vi "ES2 Main.vi"(10 "Data Type DVRs":T1, 11 "Config Folder":path) -> ()   [LabVIEW 2018]
uses:
  <vilib>/ORNL/CSEISMIC DDS/CSEISMIC DDS Base/Data Types/Controls/DeviceID.ctl
  Controls/DDS State.ctl
  Controls/Data Type DVRs.ctl
  Controls/Generation Mode Loop Selector.ctl
  <vilib>/ORNL/CSEISMIC DDS/CSEISMIC DDS Base/Data Types/DER_setGenerationMode.ctl
  <vilib>/ORNL/CSEISMIC DDS/CSEISMIC DDS Base/Data Types/Controls/Generation Mode.ctl
  Controls/GenerationMode.ctl
  <vilib>/ORNL/CSEISMIC DDS/CSEISMIC DDS Base/Data Types/IED_Status.ctl
  <vilib>/ORNL/CSEISMIC DDS/CSEISMIC DDS Base/Data Types/Controls/Timestamp.ctl
  <vilib>/ORNL/CSEISMIC DDS/CSEISMIC DDS Base/Data Types/DER_Control.ctl
  <vilib>/ORNL/CSEISMIC DDS/CSEISMIC DDS Base/Data Types/DER_SetPointP.ctl
  <vilib>/ORNL/CSEISMIC DDS/CSEISMIC DDS Base/Data Types/DER_SetPointQ.ctl
  <vilib>/ORNL/CSEISMIC DDS/CSEISMIC DDS Base/Data Types/DER_SetPointV.ctl
  <vilib>/ORNL/CSEISMIC DDS/CSEISMIC DDS Base/Data Types/DER_VF.ctl
  <vilib>/ORNL/CSEISMIC DDS/CSEISMIC DDS Base/Data Types/DER_SetPointF.ctl
  <vilib>/ORNL/CSEISMIC DDS/CSEISMIC DDS Base/Data Types/DER_Measurement.ctl
  <vilib>/ORNL/CSEISMIC DDS/CSEISMIC DDS Base/Data Types/DER_Status.ctl
  <vilib>/ORNL/CSEISMIC DDS/CSEISMIC DDS Base/Data Types/Controls/DroopCurve.ctl
  <vilib>/ORNL/CSEISMIC DDS/CSEISMIC DDS Base/Data Types/ES_Measurement.ctl
  c0909f76-96e0-496f-a6f7-ac9c3abfbcaa.vi
  7c59bdfa-a6d0-42ea-a36a-6a540bb37f3e.vi
  e95f3c18-e29d-40e4-94d7-6429cff7ece6.vi
  5e6c5b3f-77aa-4a8f-ba55-705d5b229056.vi
  7d30dc78-1fe7-43d0-be68-14ef1da03709.vi
  d3906dff-0d56-43f1-806b-b312a818046b.vi
  60710d3d-d05d-4e06-abc4-5833922697d4.vi
  d723711c-90b5-43fd-9837-430fe65d8763.vi
  2b29db2b-b629-43ef-99c9-7f779e92d8e6.vi
  fb202ae5-af77-46d5-8a34-636558cc811c.vi
  de1367b4-29ab-415d-92d0-7fa0fc6667ea.vi
  a8c78b73-a0ab-4721-a181-3ce0dcbdf431.vi
  9b782105-9e9e-450c-bef0-451d1281a5e4.vi
  04e9c7aa-85a8-4273-86f5-9355a9113040.vi
  f60448c4-0b4d-4df0-bc80-4b02817c393f.vi
  ae97810f-c92e-4387-8c39-39f975af07db.vi
  Global Variables/Stop (Global).vi
  Global Variables/Measurements (Global).vi
  Global Variables/DDS States (Global).vi
  <vilib>/ORNL/CSEISMIC DDS/CSEISMIC DDS Base/CSEISMIC DDS.lvclass
panel:
  out "P_ref":sgl
  out "Q_ref":sgl
  out "P_meas":sgl
  out "Vf Control":bool
  out "Q_meas":sgl
  out "f_islanded":fxp<+,20,6>
  out "Vq_ref":sgl
  out "5038 Count":u32
  out "Is VF Device?":bool
  in  "Ramp Rate (W)":sgl=5000.0
  out "MicrogridID":u8
  out "Error in DDS Loop":bool
  out "DDS Loop error out":errorcluster
  out "DDS State":T2=enum."Shutdown"
  out "DDS loop time":u32=103
  out "DDS Indicators":T3
  out "Error in Generation Mode Loop":bool
  out "error out GenMode Loop":errorcluster
  out "DDS state m/c loop time":u32=100
  out "DeviceID":T4
  out "Enable INV A":bool
  out "SOC":dbl
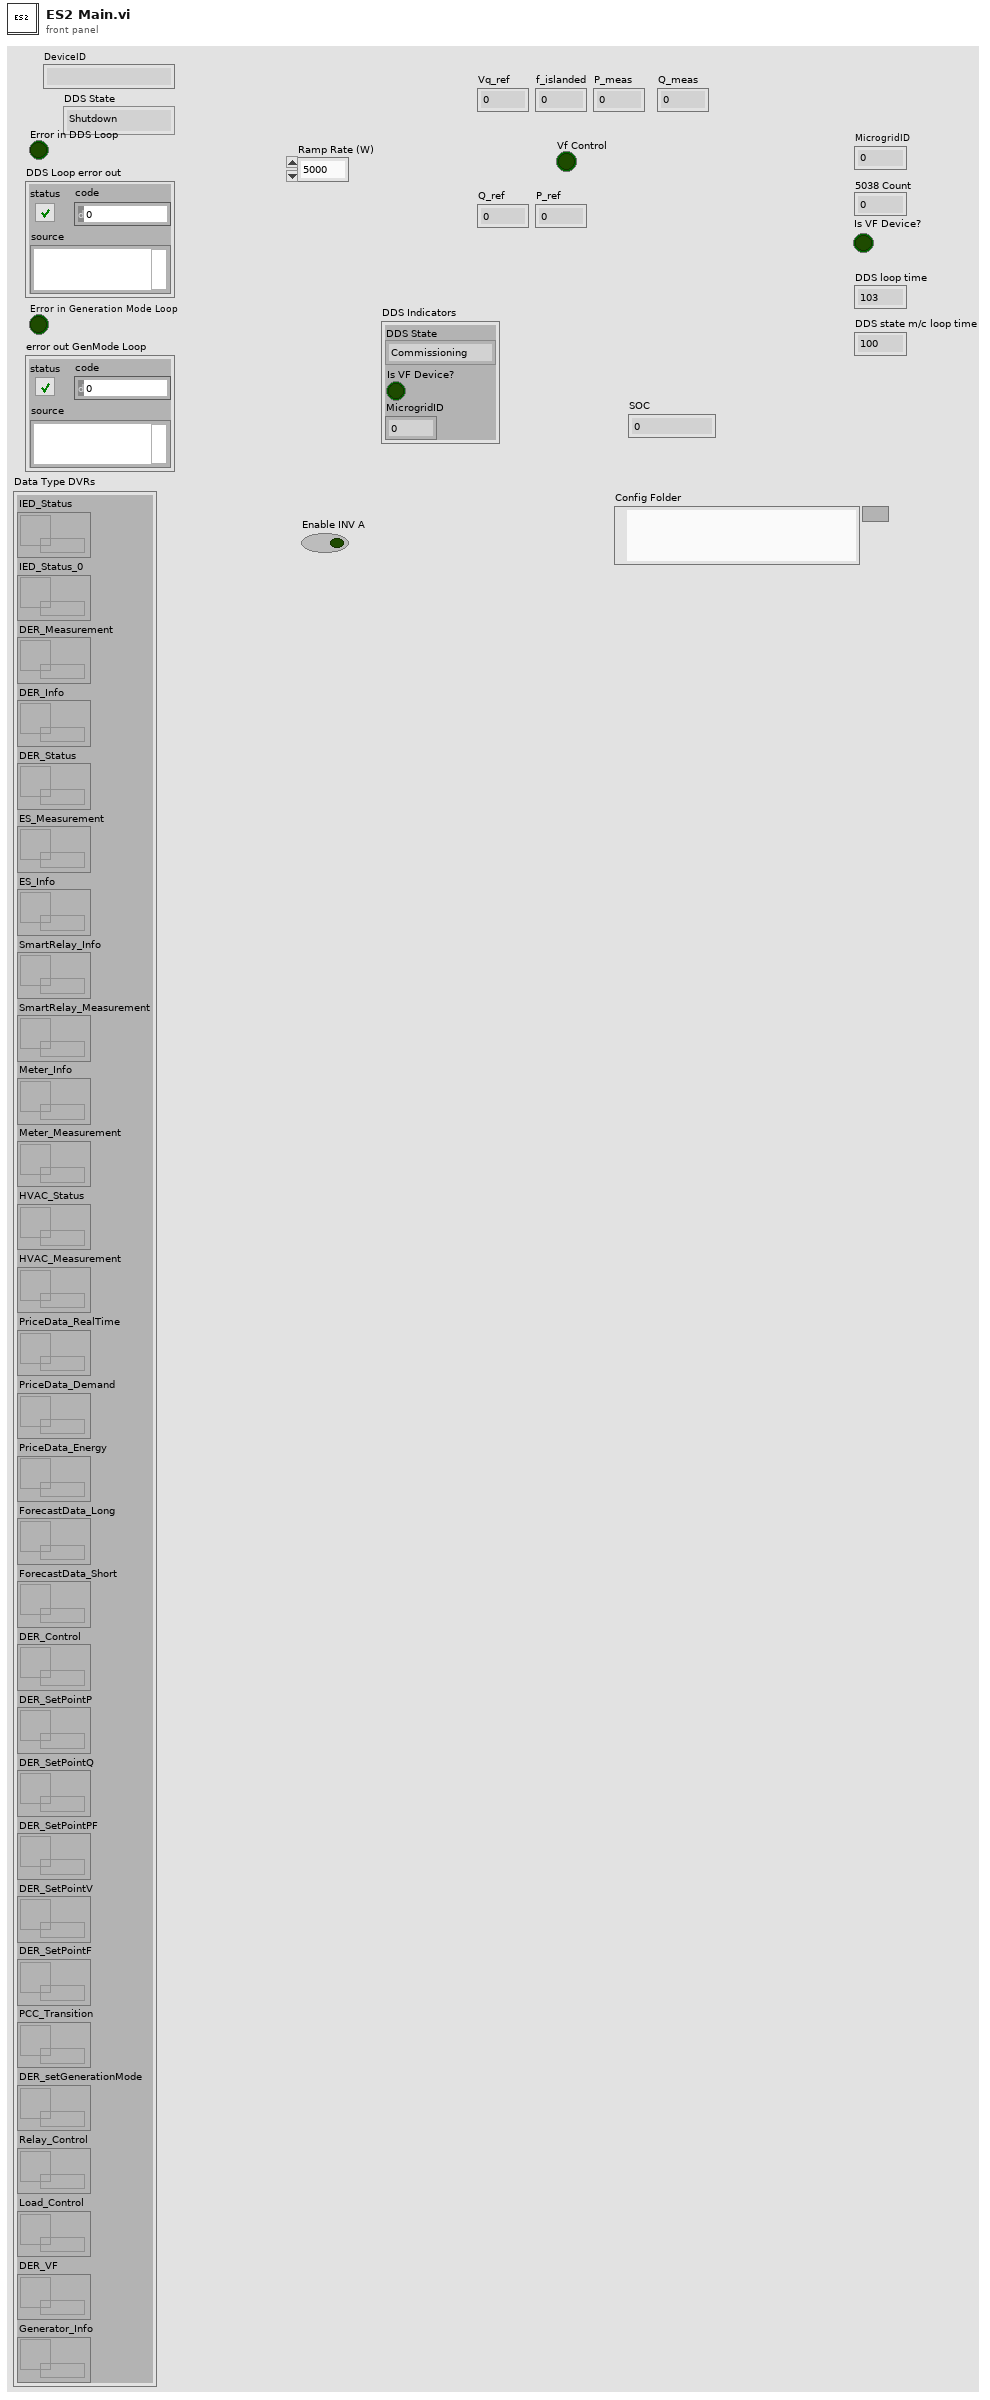
[diagram p1: front panel]
types:
  T1 = typedef "Data Type DVRs.ctl" = cluster{"IED_Status":refnum<data-value>, "IED_Status_0":refnum<data-value>, "DER_Measurement":refnum<data-value>, "DER_Info":refnum<data-value>, "DER_Status":refnum<data-value>, "ES_Measurement":refnum<data-value>, "ES_Info":refnum<data-value>, "SmartRelay_Info":refnum<data-value>, "SmartRelay_Measurement":refnum<data-value>, "Meter_Info":refnum<data-value>, "Meter_Measurement":refnum<data-value>, "HVAC_Status":refnum<data-value>, "HVAC_Measurement":refnum<data-value>, "PriceData_RealTime":refnum<data-value>, "PriceData_Demand":refnum<data-value>, "PriceData_Energy":refnum<data-value>, "ForecastData_Long":refnum<data-value>, "ForecastData_Short":refnum<data-value>, "DER_Control":refnum<data-value>, "DER_SetPointP":refnum<data-value>, "DER_SetPointQ":refnum<data-value>, "DER_SetPointPF":refnum<data-value>, "DER_SetPointV":refnum<data-value>, "DER_SetPointF":refnum<data-value>, "PCC_Transition":refnum<data-value>, "DER_setGenerationMode":refnum<data-value>, "Relay_Control":refnum<data-value>, "Load_Control":refnum<data-value>, "DER_VF":refnum<data-value>, "Generator_Info":refnum<data-value>}
  T2 = typedef "DDS State.ctl" = enum16{"Commissioning", "CheckID", "InitDDS", "ReadDDS", "WriteDDS", "CheckClose", "Close", "Shutdown"}
  T3 = cluster{"DDS State":T2, "Is VF Device?":bool, "MicrogridID":u8}
  T4 = typedef "CSEISMIC DDS.lvlib/CSEISMIC DDS.lvclass/DeviceID.ctl" = string
  T5 = typedef "Generation Mode Loop Selector.ctl" = enum16{"Commissioning", "Start", "Active", "VF Device", "Hold", "Close References", "Shutdown"}
  T6 = typedef "Scaling Coefficients Cluster.ctl" = cluster{"Measurements":T7, "Setpoints":T8}
  T7 = typedef "Scaling Coefficients Measurements.ctl" = cluster{"Current":dbl, "Voltage":dbl, "Real Power":dbl, "Reactive Power":dbl, "SOC":dbl}
  T8 = typedef "Scaling Coefficients Setpoints.ctl" = cluster{"Voltage":dbl, "Frequency":dbl, "Real Power":dbl, "Reactive Power":dbl}
  T9 = typedef "CSEISMIC DDS.lvlib/CSEISMIC DDS.lvclass/DER_Info.ctl" = cluster{"DeviceID":T4, "LineConfig":u8[], "NominalVoltage(V)":dbl, "PowerRating(kVA)":dbl, "VFControl":bool, "PControl":bool, "QControl":bool, "PFControl":bool, "PVControl":bool, "Droop":bool, "DroopConfigurable":bool, "Unbalanced":bool}
  T10 = typedef "CSEISMIC DDS.lvlib/CSEISMIC DDS.lvclass/ES_Info.ctl" = cluster{"DeviceID":T4, "EnergyRating (kWh)":dbl, "RampRate (kW/s)":dbl, "MaxPowerFactorLeading":dbl, "MaxPowerFactorLagging":dbl, "ChargingEfficiencyCurve":T11, "DischargingEfficiencyCurve":T11, "MinSOC (%)":dbl, "MaxSOC (%)":dbl}
  T11 = typedef "CSEISMIC DDS.lvlib/CSEISMIC DDS.lvclass/EfficiencyCurve.ctl" = cluster{"Power (kW)":dbl[], "Efficiency (%)":dbl[]}
  T12 = typedef "CSEISMIC DDS.lvlib/CSEISMIC DDS.lvclass/DER_setGenerationMode.ctl" = cluster{"DeviceID":T4, "Mode":T13}
  T13 = typedef "CSEISMIC DDS.lvlib/CSEISMIC DDS.lvclass/Generation Mode.ctl" = enum32{"Invalid", "PQ", "Droop", "PV", "PF", "VF"}
  T14 = typedef "GenerationMode.ctl" = enum32{"Invalid", "PQ", "Droop", "PV", "PF", "VF"}
  T15 = typedef "CSEISMIC DDS.lvlib/CSEISMIC DDS.lvclass/Timestamp.ctl" = cluster{"Seconds":u64, "Remainder":u64}
  T16 = typedef "CSEISMIC DDS.lvlib/CSEISMIC DDS.lvclass/IED_Status.ctl" = cluster{"DeviceID":T4, "Timestamp":T15, "MicrogridID":u8, "Active":bool, "Inactive":bool, "Error":i32, "Fault":bool, "ErrorString":string}
  T17 = typedef "CSEISMIC DDS.lvlib/CSEISMIC DDS.lvclass/DER_SetPointF.ctl" = cluster{"DeviceID":T4, "Frequency (Hz)":dbl}
  T18 = typedef "CSEISMIC DDS.lvlib/CSEISMIC DDS.lvclass/DER_VF.ctl" = cluster{"DeviceID":T4}
  T19 = typedef "CSEISMIC DDS.lvlib/CSEISMIC DDS.lvclass/DER_SetPointV.ctl" = cluster{"DeviceID":T4, "Voltage (V)":dbl}
  T20 = typedef "CSEISMIC DDS.lvlib/CSEISMIC DDS.lvclass/DER_SetPointQ.ctl" = cluster{"DeviceID":T4, "ReactivePower (kVAR)":dbl[]}
  T21 = typedef "CSEISMIC DDS.lvlib/CSEISMIC DDS.lvclass/DER_SetPointP.ctl" = cluster{"DeviceID":T4, "RealPower (kW)":dbl[]}
  T22 = typedef "CSEISMIC DDS.lvlib/CSEISMIC DDS.lvclass/DER_Control.ctl" = cluster{"DeviceID":T4, "Activate":bool, "Deactivate":bool}
  T23 = typedef "CSEISMIC DDS.lvlib/CSEISMIC DDS.lvclass/ES_Measurement.ctl" = cluster{"DeviceID":T4, "SOC (%)":dbl}
  T24 = typedef "CSEISMIC DDS.lvlib/CSEISMIC DDS.lvclass/DER_Status.ctl" = cluster{"DeviceID":T4, "VFControl":bool, "PControl":bool, "QControl":bool, "PFControl":bool, "PVControl":bool, "Droop":bool, "Unbalanced":bool, "MicrogridVF":bool, "RealDroop(kW)":T25, "ReactiveDroop(kVar)":T25}
  T25 = typedef "CSEISMIC DDS.lvlib/CSEISMIC DDS.lvclass/DroopCurve.ctl" = cluster{"XMin":dbl, "XMax":dbl, "YMin":dbl, "YMax":dbl}
  T26 = typedef "CSEISMIC DDS.lvlib/CSEISMIC DDS.lvclass/DER_Measurement.ctl" = cluster{"DeviceID":T4, "Voltage":dbl[], "Current":dbl[], "RealPower":dbl[], "ReactivePower":dbl[], "LineConfig":u8[], "Frequency":dbl}
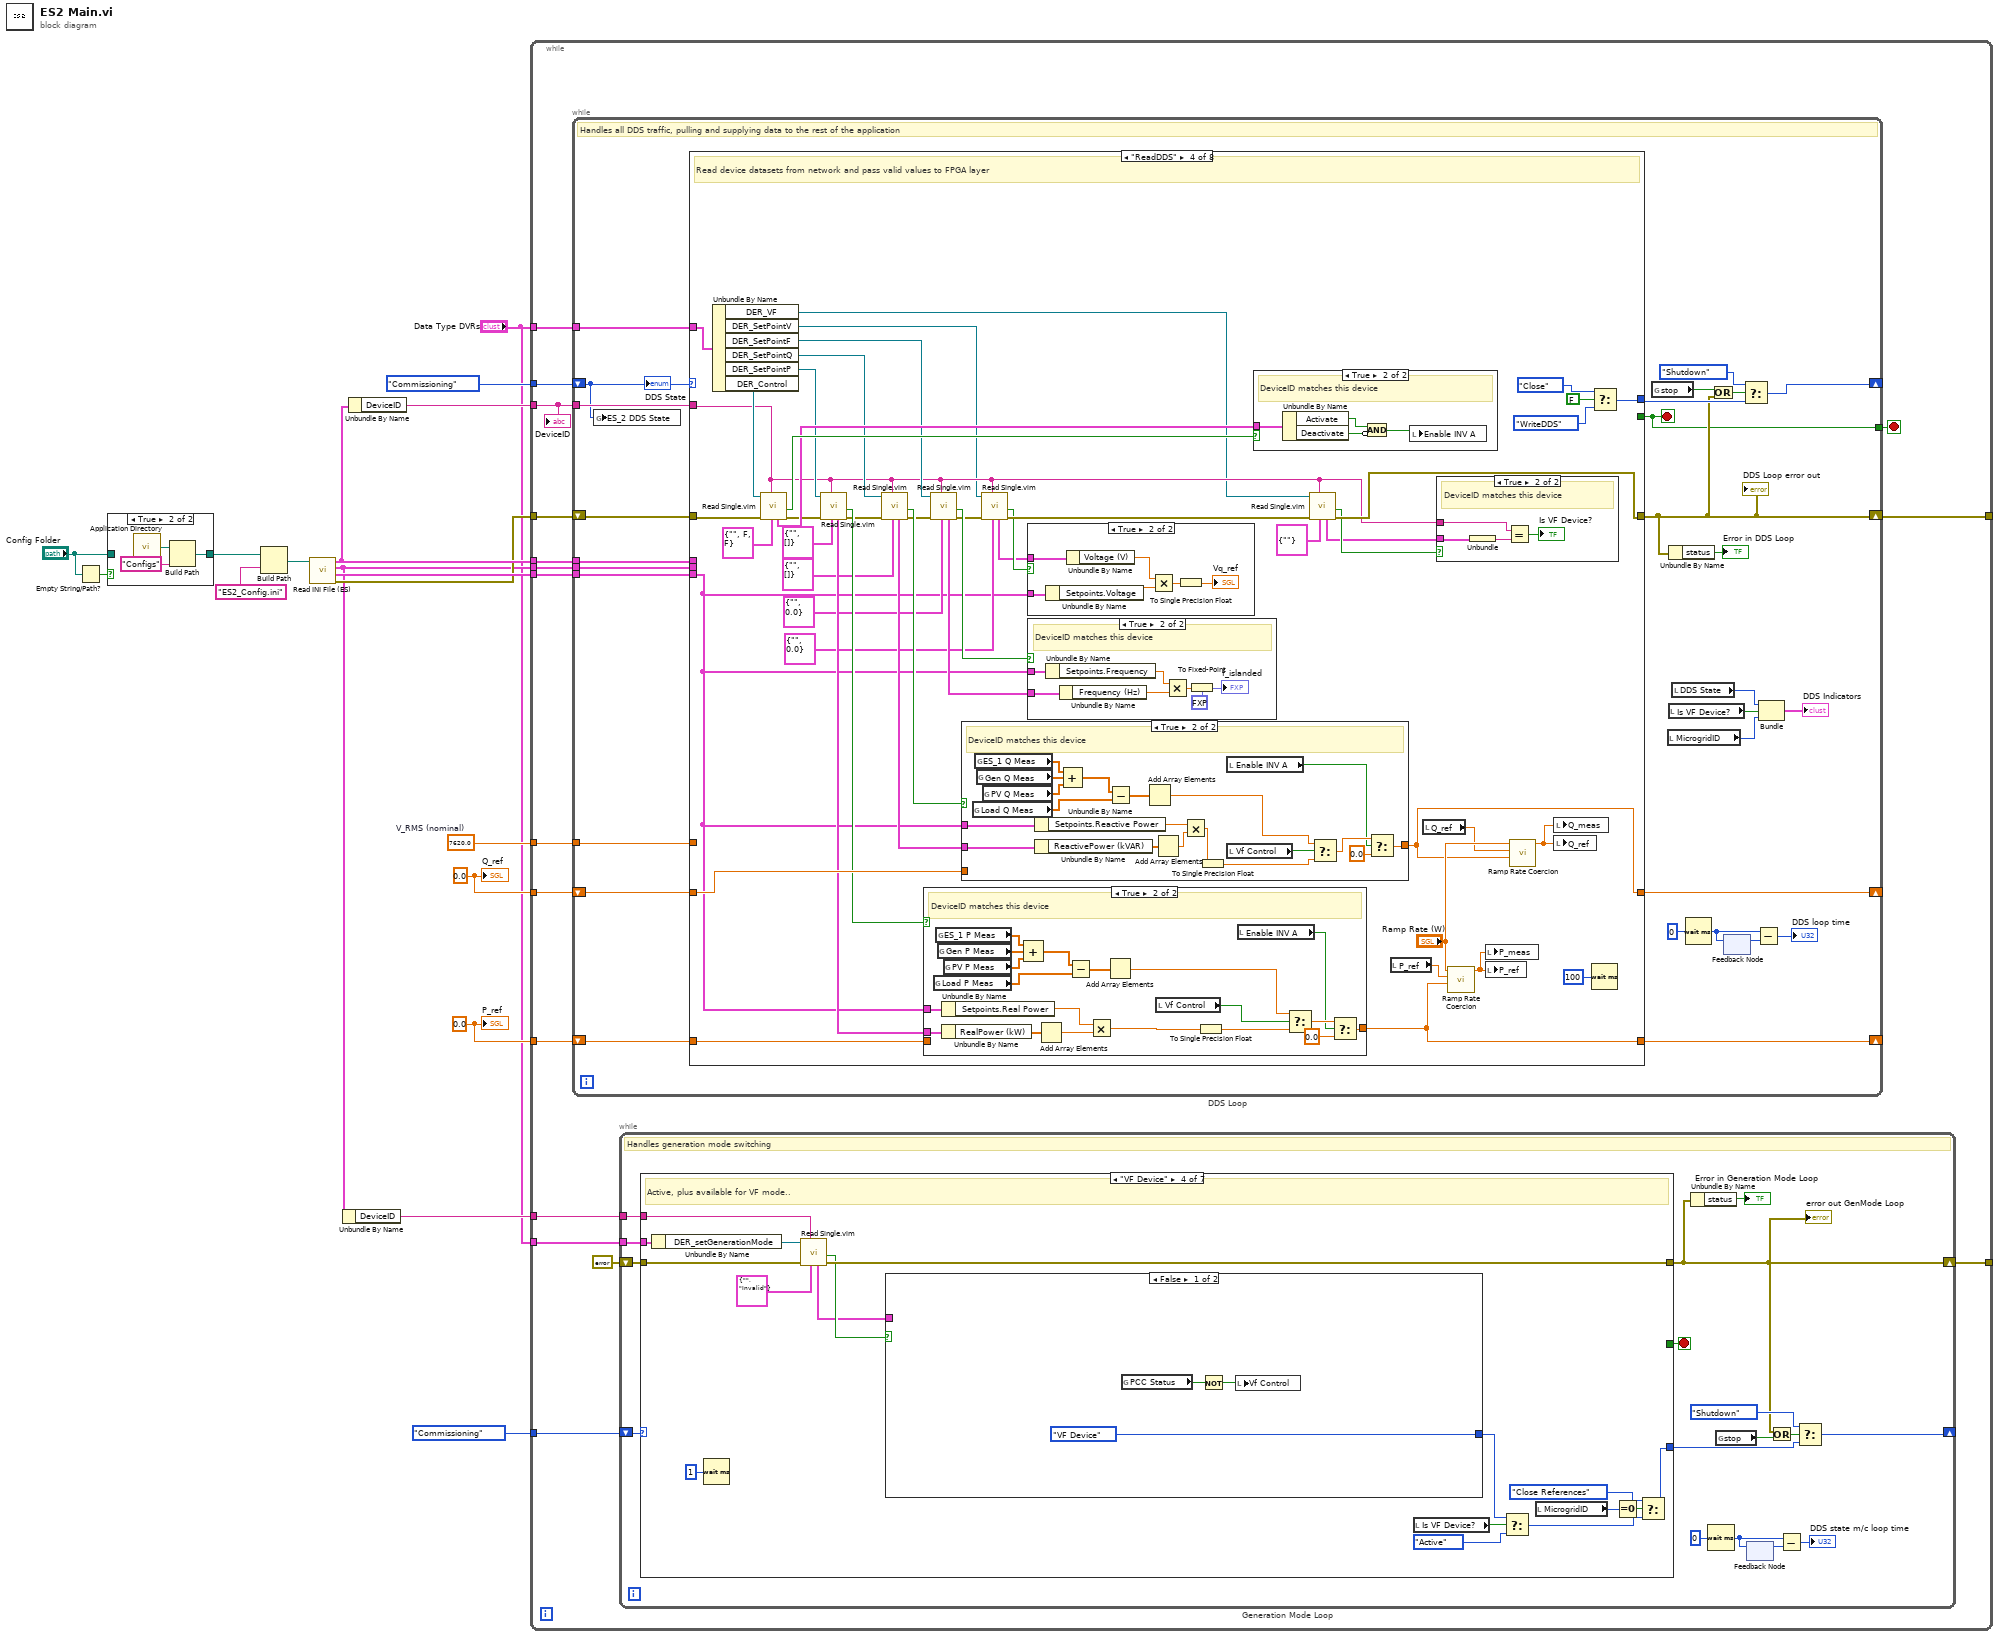
[diagram p0: block diagram]
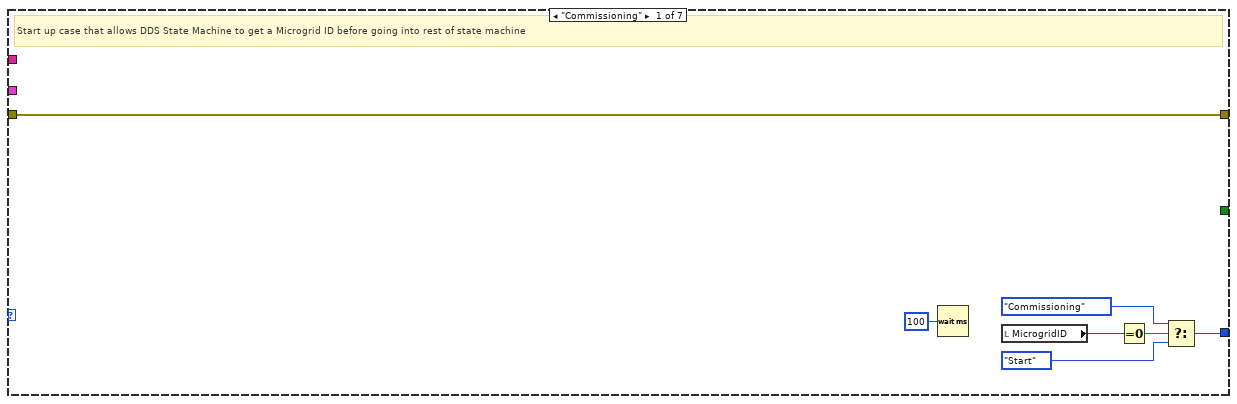
[diagram p2: hidden frame]
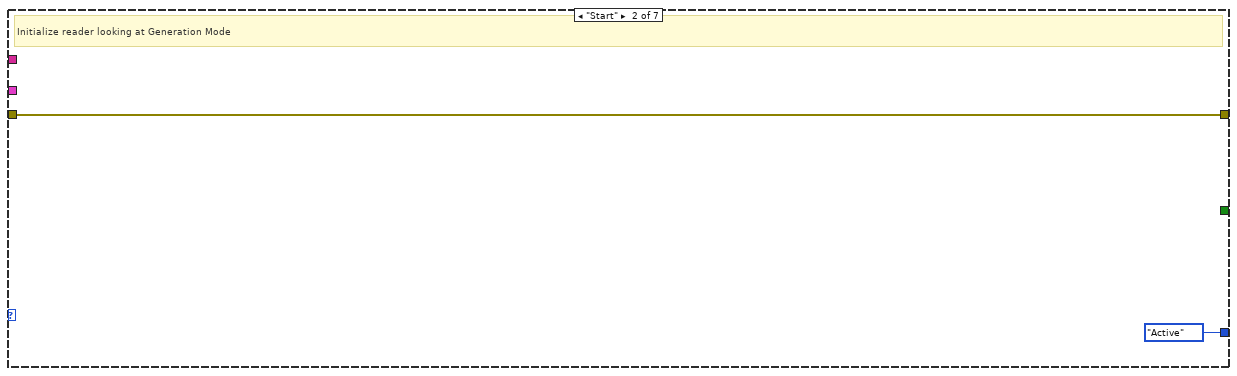
[diagram p3: hidden frame]
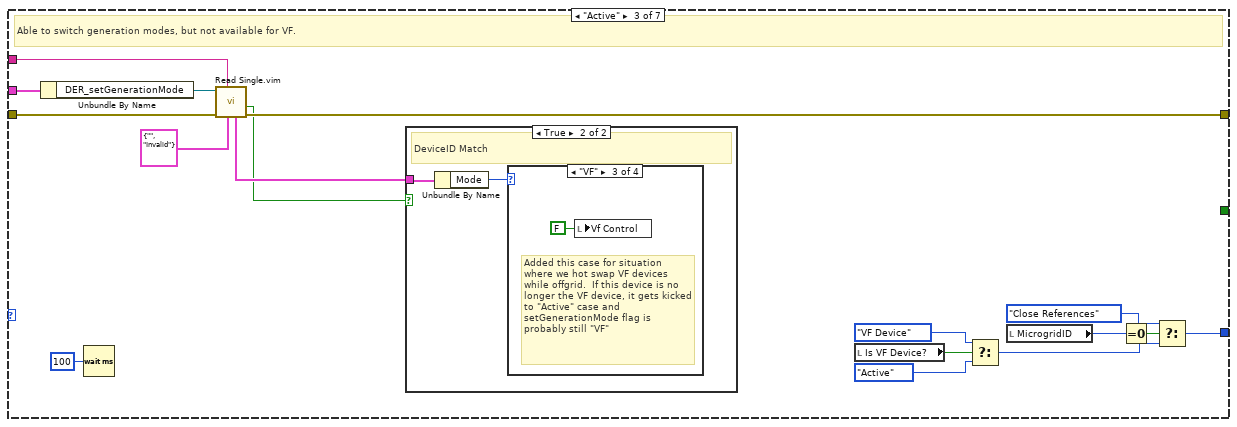
[diagram p4: hidden frame]
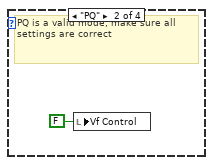
[diagram p7: hidden frame]
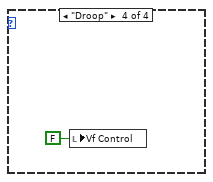
[diagram p8: hidden frame]
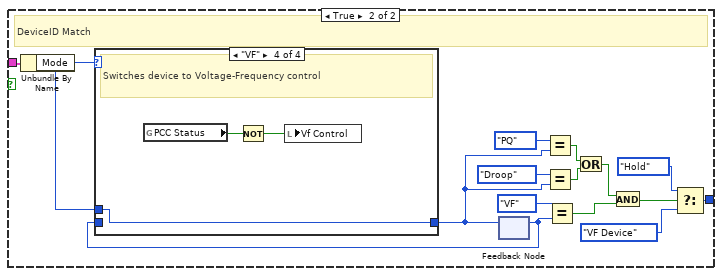
[diagram p9: hidden frame]
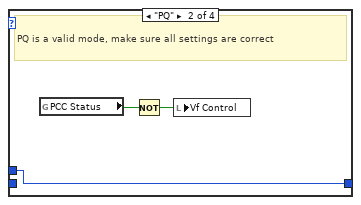
[diagram p11: hidden frame]
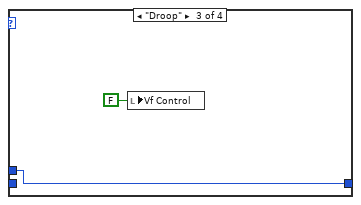
[diagram p12: hidden frame]
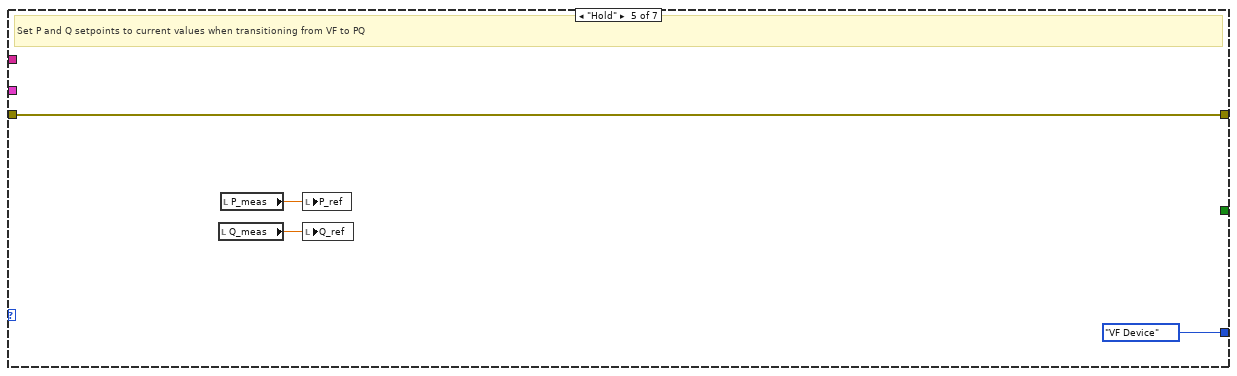
[diagram p13: hidden frame]
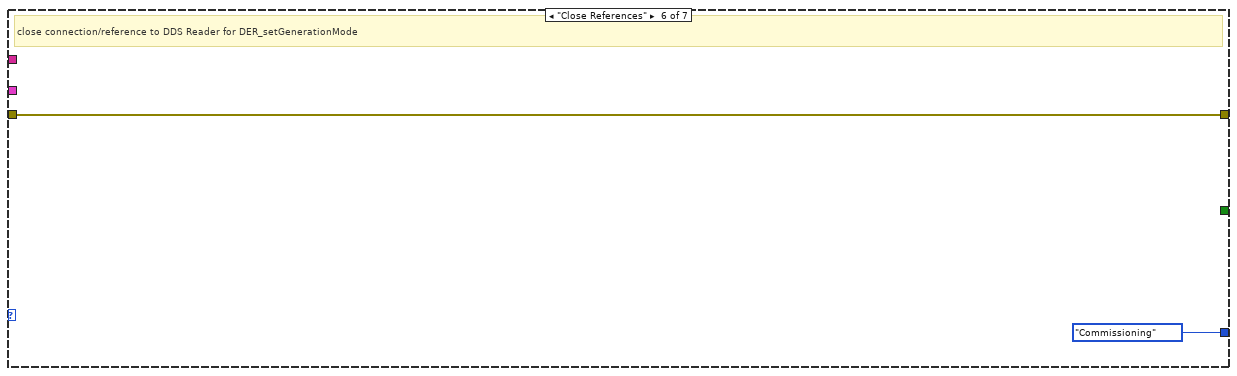
[diagram p14: hidden frame]
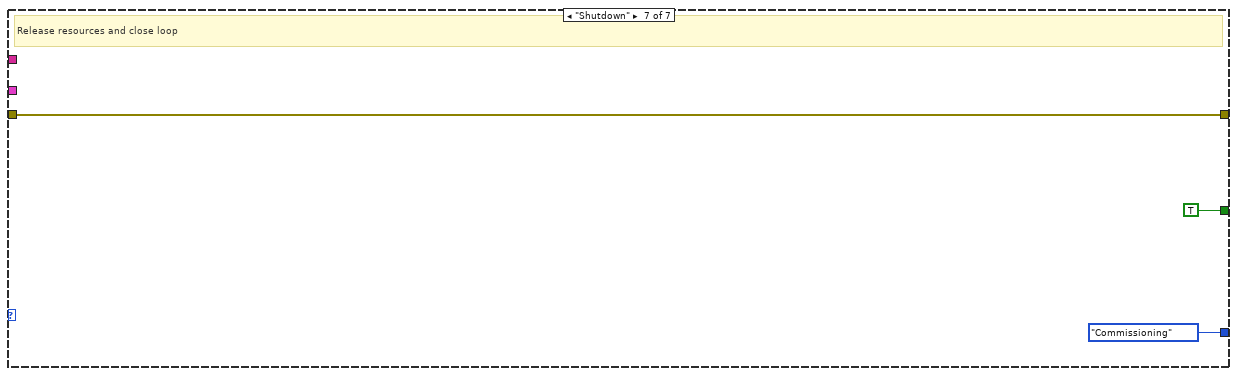
[diagram p15: hidden frame]
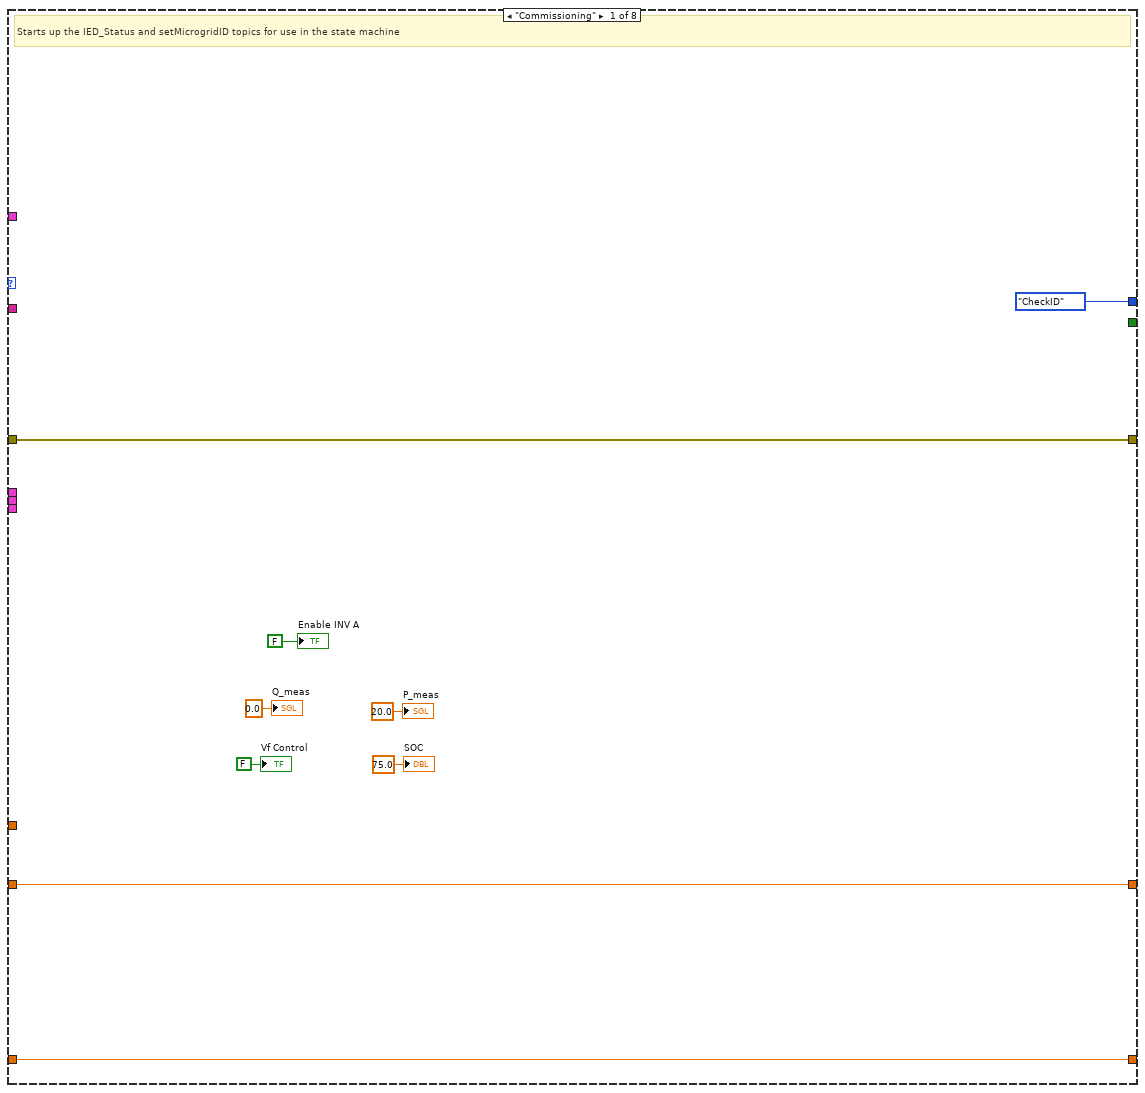
[diagram p16: hidden frame]
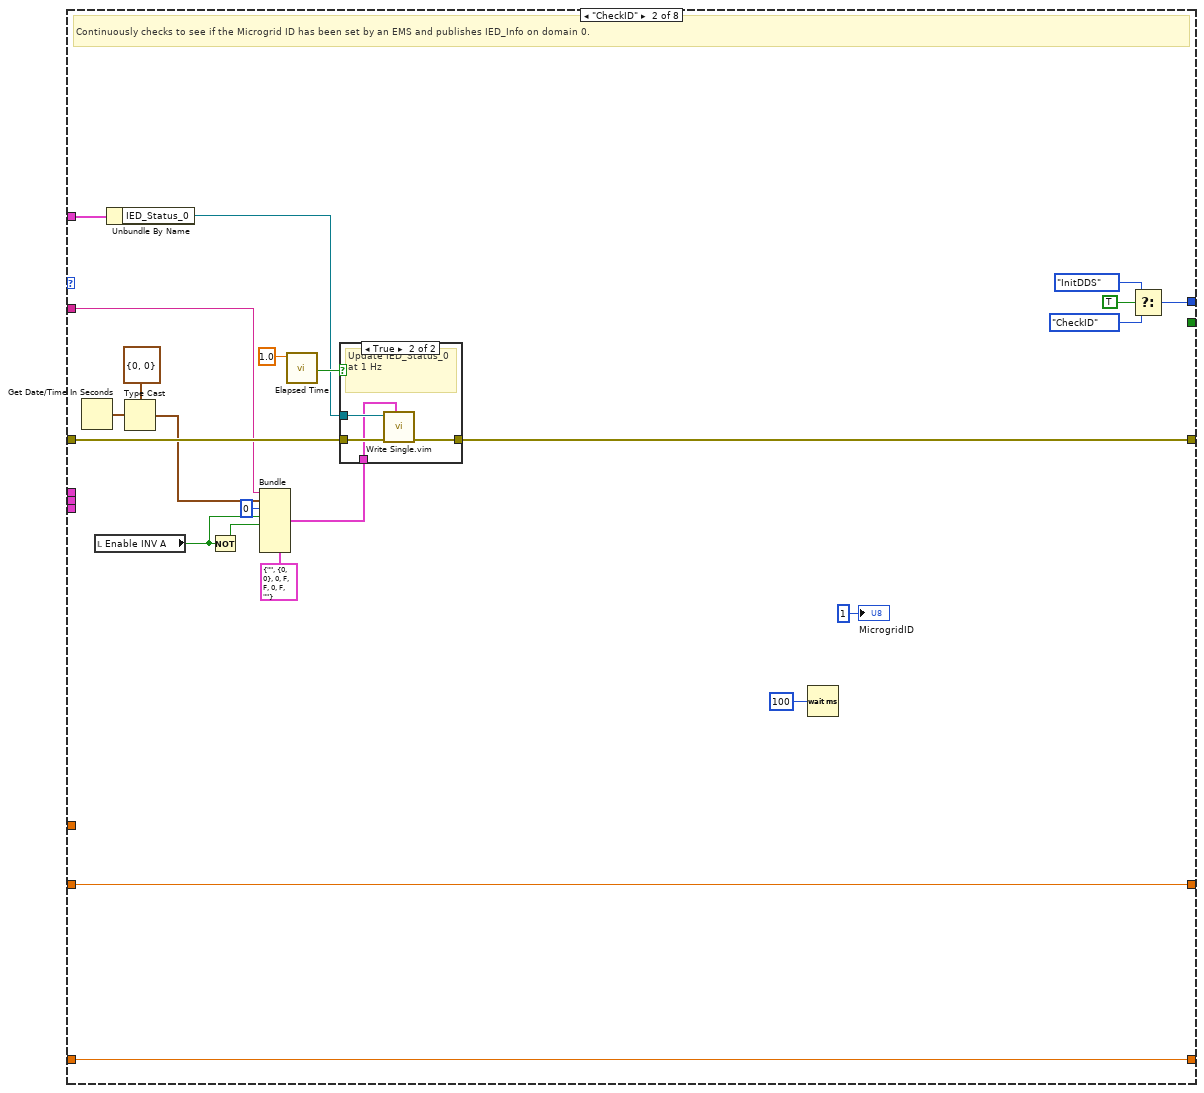
[diagram p17: hidden frame]
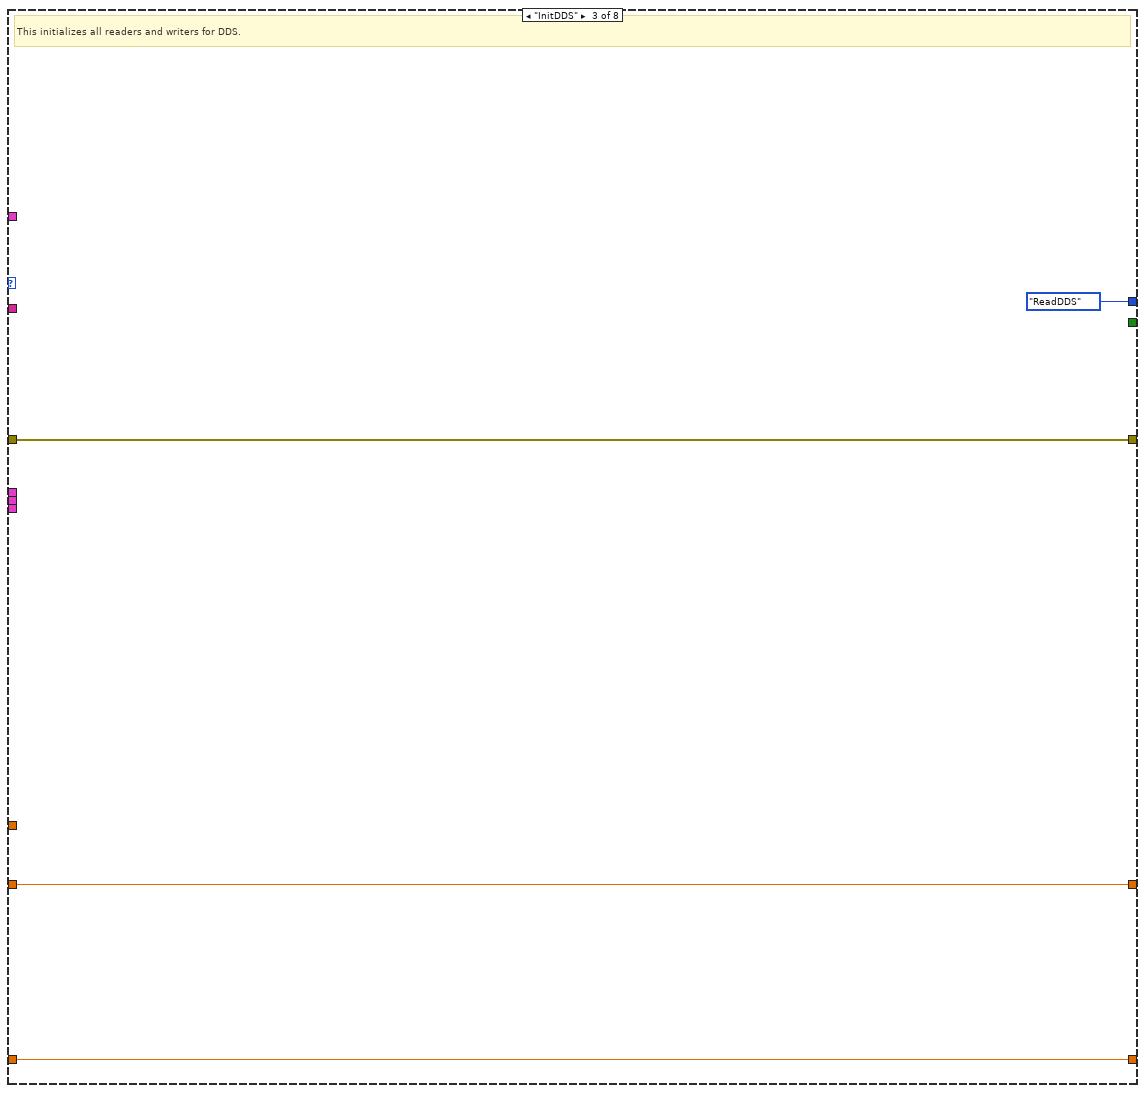
[diagram p19: hidden frame]
diagram:
  w5 = 7620.0  # V_RMS (nominal)
  w6 = sgl 0.0 ("Q_ref")
  w7 = sgl 0.0 ("P_ref")
  n1 = Empty String/Path?(string/path="Config Folder") -> (empty?=w4:bool)
  n2 = case shown="True" w4 {
    tunnel: [w18 w19] -> w2
    tunnel: "Config Folder" -> [w18 _]
    frame False {
    }
    frame True {
      n3 = call <vilib>:"Application Directory.vi"() -> ("Application Directory"=w21:path)
      n4 = Build Path(base path=w21, name or relative path="Configs") -> (appended path=w19:path)
    }
  }
  n5 = Build Path(base path=w2, name or relative path="ES2_Config.ini") -> (appended path=w16:path)
  n6 = call "Read INI File (ES).vi"("Path"=w16) -> ("error out"=w12:errorcluster, "Scaling Coefficients"=w13:T6, "DER_Info"=w10:T9, "ES_Info"=w14:T10)  [unwired: 7 in]
  n7 = Unbundle By Name(w10) -> ("DeviceID"=w11:T4)
  n8 = Unbundle By Name(w14) -> ("DeviceID"=w15:T4)
  n9 = while {
    tunnel: DDS_State."Commissioning" ("DDS State 2") -> [w38]
    tunnel: w10 -> [w37]
    tunnel: w12 -> [w36]
    tunnel: w13 -> [w35]
    tunnel: w15 -> [w34]
    tunnel: w14 -> [w33]
    tunnel: w11 -> [w31]
    tunnel: Generation_Mode_Loop_Selector."Commissioning" -> [w30]
    tunnel: [w29] -> _
    tunnel: [w28] -> _
    tunnel: w7 -> [w27]
    tunnel: w6 -> [w26]
    tunnel: w5 -> [w25]
    tunnel: "Data Type DVRs" -> [w24]
    tunnel: "Data Type DVRs" -> [w23]
    stop <- w32 stop-if-true
    n10 = while "DDS Loop" {
      shift-right: [w162] -> _
      shift-left: w38 -> [w139]
      tunnel: w34 -> [w166]
      shift-right: [w157] -> w28
      shift-left: w36 -> [w165]
      tunnel: w33 -> [w164]
      tunnel: w37 -> [w163]
      tunnel: w35 -> [w158]
      tunnel: [w155] -> w32
      shift-right: [w149] -> _
      shift-left: w27 -> [w148]
      shift-right: [w147] -> _
      shift-left: w26 -> [w146]
      tunnel: w25 -> [w141]
      tunnel: w24 -> [w150]
      stop <- w155 stop-if-true
      # "Handles all DDS traffic, pulling and supplying data to the rest of the application"
      n11 = global write "DDS States (Global).vi" "ES_2 DDS State"(w139) -> ()
      n12 = case shown="\"ReadDDS\"" w139 {
        tunnel: [DDS_State."CheckID" w193 DDS_State."ReadDDS" w253 DDS_State."CheckClose" w437 DDS_State."Commissioning" ("f") DDS_State."Commissioning" ("f")] -> w161
        tunnel: [w174 w184 w206 w220 w366 w436 w443 w450] -> w157
        tunnel: w166 -> [_ w183 _ w217 w351 _ _ _]
        tunnel: w165 -> [w174 w196 w206 w240 w385 w436 w443 w450]
        tunnel: w164 -> [_ _ _ _ w377 _ _ _]
        tunnel: w163 -> [_ _ _ _ w376 _ _ _]
        tunnel: [_ _ _ _ _ _ _ TRUE] -> w155
        tunnel: w158 -> [_ _ _ w209 w372 _ _ _]
        tunnel: w150 -> [_ w178 _ w241 w325 _ _ _]
        tunnel: [w173 w182 w205 w251 w344 w435 w441 w447] -> w149
        tunnel: w148 -> [w173 w182 w205 w250 w344 w435 w441 w447]
        tunnel: [w172 w181 w204 w248 w343 w434 w440 w446] -> w147
        tunnel: w146 -> [w172 w181 w204 w247 w343 w434 w440 w446]
        tunnel: w141 -> [_ _ _ _ w333 _ _ _]
        frame "Commissioning" {
          # "Starts up the IED_Status and setMicrogridID topics for use in the state machine"
          "Q_meas" <- sgl 0.0 ("Q_meas")
          "Vf Control" <- FALSE ("Vf Control")
          "P_meas" <- sgl 20.0 ("P_meas")
          "SOC" <- 75.0 ("SOC")
          "Enable INV A" <- FALSE ("Enable INV A")
        }
        frame "CheckID" {
          # "Continuously checks to see if the Microgrid ID has been set by an EMS and publishes IED_Info on domain 0."
          n13 = Get Date/Time In Seconds() -> (seconds since 1Jan1904=w189:timestamp)
          n14 = local read "Enable INV A"() -> (w180:bool)
          n15 = Unbundle By Name(w178) -> ("IED_Status_0"=w177:refnum<data-value>)
          n16 = Type Cast(type=T15 {"Seconds"=0, "Remainder"=0} ("Timestamp"), x=w189) -> (*(type *) &x=w187:T15)
          n17 = Not(x=w180) -> (.not. x?=w185:bool)
          n18 = Bundle(cluster=T16 {"DeviceID"="", "Timestamp"={"Seconds"=0, "Remainder"=0}, "MicrogridID"=0, "Active"=FALSE, "Inactive"=FALSE, "Error"=0, "Fault"=FALSE, "ErrorString"=""} ("output cluster"), "DeviceID"=w183, "Timestamp"=w187, "MicrogridID"=u8 0, "Active"=w180, "Inactive"=w185) -> (w197:T16)  [unwired: 3 in]
          n19 = call "Elapsed Time"("Time Target (s)"=1.0) -> ("Time has Elapsed"=w192:bool)  [unwired: 11 in, 7 out]
          n20 = case shown="True" w192 {
            tunnel: w197 -> [_ w200]
            tunnel: [w199 w201] -> w184
            tunnel: w196 -> [w199 w202]
            tunnel: w177 -> [_ w203]
            frame False {
            }
            frame True {
              # "Update IED_Status_0 at 1 Hz"
              n21 = call "Write Single.vim"("Data Element"=w200, "error in"=w202, "Data DVR"=w203) -> ("dup error out"=w201:errorcluster)  [unwired: 8 in]
            }
          }
          n22 = Wait (ms)(milliseconds to wait=u32 100) -> ()  [unwired: 1 out]
          n23 = Select(t=DDS_State."InitDDS", s=TRUE, f=DDS_State."CheckID") -> (s? t:f=w193:T2)
          "MicrogridID" <- u8 1 ("MicrogridID")
        }
        frame "InitDDS" {
          # "This initializes all readers and writers for DDS."
        }
        frame "ReadDDS" {
          # "Read device datasets from network and pass valid values to FPGA layer"
          n24 = Unbundle By Name(w241) -> ("DER_VF"=w216:refnum<data-value>, "DER_SetPointV"=w214:refnum<data-value>, "DER_SetPointF"=w225:refnum<data-value>, "DER_SetPointQ"=w229:refnum<data-value>, "DER_SetPointP"=w233:refnum<data-value>, "DER_Control"=w239:refnum<data-value>)
          n25 = call "Read Single.vim"("Data Type"=T22 {"DeviceID"="", "Activate"=FALSE, "Deactivate"=FALSE} ("DER_Control"), "DeviceID"=w217, "error in"=w240, "Data DVR"=w239) -> ("dup error out"=w235:errorcluster, "Valid"=w238:bool, "Data Element"=w237:T22)  [unwired: 5 in]
          n26 = call "Read Single.vim"("Data Type"=T21 {"DeviceID"="", "RealPower (kW)"=[]} ("DER_SetPointP"), "DeviceID"=w217, "error in"=w235, "Data DVR"=w233) -> ("dup error out"=w230:errorcluster, "Valid"=w232:bool, "Data Element"=w231:T21)  [unwired: 5 in]
          n27 = call "Read Single.vim"("Data Type"=T20 {"DeviceID"="", "ReactivePower (kVAR)"=[]} ("DER_SetPointQ"), "DeviceID"=w217, "error in"=w230, "Data DVR"=w229) -> ("dup error out"=w224:errorcluster, "Valid"=w227:bool, "Data Element"=w226:T20)  [unwired: 5 in]
          n28 = case shown="True" w232 {
            tunnel: w231 -> [_ w313]
            tunnel: w209 -> [_ w312]
            tunnel: [w294 w307] -> w251
            tunnel: w250 -> [w294 _]
            frame False {
              # "Non-matching DeviceID"
            }
            frame True {
              # "DeviceID matches this device"
              n29 = global read "Measurements (Global).vi" "Load P Meas"() -> (w300:dbl[])
              n30 = global read "Measurements (Global).vi" "ES_1 P Meas"() -> (w296:dbl[])
              n31 = global read "Measurements (Global).vi" "Gen P Meas"() -> (w297:dbl[])
              n32 = Unbundle By Name(w312) -> ("Setpoints.Real Power"=w310:dbl)
              n33 = Unbundle By Name(w313) -> ("RealPower (kW)"=w311:dbl[])
              n34 = global read "Measurements (Global).vi" "PV P Meas"() -> (w298:dbl[])
              n35 = Compound Arithmetic op=ADD(w296, w297, w298) -> (w299:dbl[])
              n36 = Add Array Elements(numeric array=w311) -> (sum=w309:dbl)
              n37 = Subtract(x=w299, y=w300) -> (x-y=w301:dbl[])
              n38 = Multiply(x=w310, y=w309) -> (x*y=w308:dbl)
              n39 = Add Array Elements(numeric array=w301) -> (sum=w295:dbl)
              n40 = local read "Vf Control"() -> (w303:bool)
              n41 = To Single Precision Float(number=w308) -> (single precision float=w305:sgl)
              n42 = local read "Enable INV A"() -> (w302:bool)
              n43 = Select(t=w295, s=w303, f=w305) -> (s? t:f=w304:dbl)
              n44 = Select(t=w304, s=w302, f=sgl 0.0) -> (s? t:f=w307:dbl)
            }
          }
          n45 = call "Read Single.vim"("Data Type"=T17 {"DeviceID"="", "Frequency (Hz)"=0.0} ("DER_SetPointVF"), "DeviceID"=w217, "error in"=w224, "Data DVR"=w225) -> ("dup error out"=w213:errorcluster, "Valid"=w223:bool, "Data Element"=w222:T17)  [unwired: 5 in]
          n46 = case shown="True" w227 {
            tunnel: w226 -> [_ w293]
            tunnel: w209 -> [_ w292]
            tunnel: [w274 w284] -> w248
            tunnel: w247 -> [w274 _]
            frame False {
              # "Non-matching DeviceID"
            }
            frame True {
              # "DeviceID matches this device"
              n47 = global read "Measurements (Global).vi" "Load Q Meas"() -> (w277:dbl[])
              n48 = global read "Measurements (Global).vi" "ES_1 Q Meas"() -> (w281:dbl[])
              n49 = global read "Measurements (Global).vi" "Gen Q Meas"() -> (w280:dbl[])
              n50 = global read "Measurements (Global).vi" "PV Q Meas"() -> (w279:dbl[])
              n51 = Unbundle By Name(w292) -> ("Setpoints.Reactive Power"=w289:dbl)
              n52 = Unbundle By Name(w293) -> ("ReactivePower (kVAR)"=w291:dbl[])
              n53 = Compound Arithmetic op=ADD(w281, w280, w279) -> (w278:dbl[])
              n54 = Subtract(x=w278, y=w277) -> (x-y=w276:dbl[])
              n55 = Add Array Elements(numeric array=w276) -> (sum=w275:dbl)
              n56 = Add Array Elements(numeric array=w291) -> (sum=w290:dbl)
              n57 = Multiply(x=w289, y=w290) -> (x*y=w288:dbl)
              n58 = To Single Precision Float(number=w288) -> (single precision float=w287:sgl)
              n59 = local read "Enable INV A"() -> (w283:bool)
              n60 = local read "Vf Control"() -> (w282:bool)
              n61 = Select(t=w275, s=w282, f=w287) -> (s? t:f=w286:dbl)
              n62 = Select(t=w286, s=w283, f=sgl 0.0) -> (s? t:f=w284:dbl)
            }
          }
          n63 = call "Read Single.vim"("Data Type"=T19 {"DeviceID"="", "Voltage (V)"=0.0} ("DER_SetPointVF"), "DeviceID"=w217, "error in"=w213, "Data DVR"=w214) -> ("dup error out"=w212:errorcluster, "Valid"=w210:bool, "Data Element"=w208:T19)  [unwired: 5 in]
          n64 = case shown="True" w210 {
            tunnel: w209 -> [_ w259]
            tunnel: w208 -> [_ w258]
            frame False {
            }
            frame True {
              n65 = Unbundle By Name(w259) -> ("Setpoints.Voltage"=w256:dbl)
              n66 = Unbundle By Name(w258) -> ("Voltage (V)"=w257:dbl)
              n67 = Multiply(x=w257, y=w256) -> (x*y=w261:dbl)
              n68 = To Single Precision Float(number=w261) -> (single precision float=→"Vq_ref":sgl)
            }
          }
          n69 = case shown="True" w223 {
            tunnel: w222 -> [_ w273]
            tunnel: w209 -> [_ w272]
            frame False {
              # "Non-matching DeviceID"
            }
            frame True {
              # "DeviceID matches this device"
              n70 = Unbundle By Name(w272) -> ("Setpoints.Frequency"=w271:dbl)
              n71 = Unbundle By Name(w273) -> ("Frequency (Hz)"=w267:dbl)
              n72 = Multiply(x=w271, y=w267) -> (x*y=w269:dbl)
              n73 = To Fixed-Point(fixed-point type=fxp<+,20,6> 0.0 ("f_islanded"), number=w269) -> (fixed-point=→"f_islanded":fxp<+,20,6>)
            }
          }
          n74 = case shown="True" w238 {
            tunnel: w237 -> [_ w317]
            frame False {
              # "Non-matching DeviceID"
            }
            frame True {
              # "DeviceID matches this device"
              n75 = Unbundle By Name(w317) -> ("Activate"=w315:bool, "Deactivate"=w316:bool)
              n76 = Compound Arithmetic op=AND(w315, invert w316) -> (w314:bool)
              n77 = local write "Enable INV A"(w314) -> ()
            }
          }
          n78 = call "Read Single.vim"("Data Type"=T18 {"DeviceID"=""} ("DER_VF"), "DeviceID"=w217, "error in"=w212, "Data DVR"=w216) -> ("dup error out"=w220:errorcluster, "Valid"=w219:bool, "Data Element"=w218:T18)  [unwired: 5 in]
          n79 = local read "P_ref"() -> (w245:sgl)
          n80 = local read "Q_ref"() -> (w246:sgl)
          n81 = case shown="True" w219 {
            tunnel: w218 -> [_ w266]
            tunnel: w217 -> [_ w264]
            frame False {
              # "Non-matching DeviceID"
              n82 = local write "Is VF Device?"(FALSE ("Is VF Device?")) -> ()
            }
            frame True {
              # "DeviceID matches this device"
              n83 = Unbundle(w266) -> ("DeviceID"=w265:T4)
              n84 = Equal?(x=w264, y=w265) -> (x = y?=→"Is VF Device?":bool)
            }
          }
          n85 = call "Ramp Rate Coercion.vi"("Requested Value"=w251, "Original Value"=w245, "Ramp Rate (W)"="Ramp Rate (W)") -> ("Coerced Value"=w244:sgl)  [unwired: 8 in]
          n86 = local write "P_meas"(w244) -> ()
          n87 = local write "P_ref"(w244) -> ()
          n88 = call "Ramp Rate Coercion.vi"("Requested Value"=w248, "Original Value"=w246, "Ramp Rate (W)"="Ramp Rate (W)") -> ("Coerced Value"=w243:sgl)  [unwired: 8 in]
          n89 = local write "Q_meas"(w243) -> ()
          n90 = local write "Q_ref"(w243) -> ()
          n91 = Wait (ms)(milliseconds to wait=u32 100) -> ()  [unwired: 1 out]
          n92 = Select(t=DDS_State."Close", s=FALSE, f=DDS_State."WriteDDS") -> (s? t:f=w253:T2)
        }
        frame "WriteDDS" {
          w347 = sgl 3.0 ("y")
          w336 = FALSE ("PFControl")
          # "#TODO add noise"
          # "Publish required datasets at required update rates to network"
          n93 = local read "Is VF Device?"() -> (w334:bool)
          n94 = Unbundle By Name(w325) -> ("DER_Status"=w318:refnum<data-value>, "DER_Measurement"=w319:refnum<data-value>, "ES_Measurement"=w320:refnum<data-value>, "IED_Status"=w321:refnum<data-value>, "IED_Status_0"=w322:refnum<data-value>, "ES_Info"=w323:refnum<data-value>, "DER_Info"=w324:refnum<data-value>)
          n95 = Unbundle By Name(w376) -> ("LineConfig"=w375:u8[])
          n96 = Get Date/Time In Seconds() -> (seconds since 1Jan1904=w360:timestamp)
          n97 = local read "MicrogridID"() -> (w356:u8)
          n98 = Type Cast(type=T15 {"Seconds"=0, "Remainder"=0} ("Timestamp"), x=w360) -> (*(type *) &x=w357:T15)
          n99 = for {
            N: 3 -> [_]
            tunnel: [w397] -> w371 mode=indexing
            tunnel: [w396] -> w370 mode=indexing
            tunnel: w334 -> [w393]
            tunnel: w333 -> [w392]
            tunnel: [w391] -> w332
            # "#TODO add noise"
            n100 = case shown="True" w393 {
              tunnel: [w401 w406] -> w395
              tunnel: [w402 w407] -> w394
              tunnel: w392 -> [w401 _]
              tunnel: [fxp<+,20,6> 60.0 ("f_islanded") w405] -> w390
              frame False {
                n101 = local read "P_meas"() -> (w399:sgl)
                n102 = expression code="x*1000"(w399) -> (w398:sgl)
                n103 = Divide(x=w398, y=w401) -> (x/y=w402:dbl)
              }
              frame True {
                n104 = local read "P_meas"() -> (w404:sgl)
                n105 = local read "Vq_ref"() -> (w406:sgl)
                n106 = local read "f_islanded"() -> (w405:fxp<+,20,6>)
                n107 = expression code="x*1000"(w404) -> (w403:sgl)
                n108 = Divide(x=w403, y=w406) -> (x/y=w407:sgl)
              }
            }
            n109 = To Double Precision Float(number=w390) -> (double precision float=w391:dbl)
            n110 = To Double Precision Float(number=w395) -> (double precision float=w397:dbl)
            n111 = To Double Precision Float(number=w394) -> (double precision float=w396:dbl)
          }
          n112 = call "Elapsed Time4"("Time Target (s)"=1.0) -> ("Time has Elapsed"=w373:bool)  [unwired: 11 in, 7 out]
          n113 = Unbundle By Name(w372) -> ("Measurements.SOC"=w348:dbl, "Measurements.Current"=w368:dbl, "Measurements.Voltage"=w369:dbl)  [unwired: 2 out]
          n114 = local read "Enable INV A"() -> (w341:bool)
          n115 = local read "Q_meas"() -> (w339:sgl)
          n116 = local read "P_meas"() -> (w340:sgl)
          n117 = Not(x=w341) -> (.not. x?=w355:bool)
          n118 = local read "SOC"() -> (w342:dbl)
          n119 = Bundle(cluster=T16 {"DeviceID"="", "Timestamp"={"Seconds"=0, "Remainder"=0}, "MicrogridID"=0, "Active"=FALSE, "Inactive"=FALSE, "Error"=0, "Fault"=FALSE, "ErrorString"=""} ("IED_Status"), "DeviceID"=w351, "Timestamp"=w357, "MicrogridID"=w356, "Active"=w341, "Inactive"=w355) -> (w383:T16)  [unwired: 3 in]
          n120 = Divide(x=w340, y=w347) -> (x/y=w346:sgl)
          n121 = Divide(x=w339, y=w347) -> (x/y=w345:sgl)
          n122 = Multiply(x=w342, y=w348) -> (x*y=w349:dbl)
          n123 = Multiply(x=w369, y=w371) -> (x*y=w331:dbl[])
          n124 = Multiply(x=w368, y=w370) -> (x*y=w330:dbl[])
          n125 = Build Array(w346, w346, w346) -> (w329:sgl[])
          n126 = Build Array(w345, w345, w345) -> (w328:sgl[])
          n127 = To Double Precision Float(number=w329) -> (double precision float=w326:dbl[])
          n128 = To Double Precision Float(number=w328) -> (double precision float=w327:dbl[])
          n129 = call "Elapsed Time3"("Time Target (s)"=0.1) -> ("Time has Elapsed"=w378:bool)  [unwired: 11 in, 7 out]
          n130 = Bundle(cluster=T26 {"DeviceID"="", "Voltage"=[], "Current"=[], "RealPower"=[], "ReactivePower"=[], "LineConfig"=[], "Frequency"=0.0} ("DER_Measurement"), "DeviceID"=w351, "Voltage"=w331, "Current"=w330, "RealPower"=w326, "ReactivePower"=w327, "LineConfig"=w375, "Frequency"=w332) -> (w382:T26)
          n131 = local read "Vf Control"() -> (w338:bool)
          n132 = feedback #1() -> (w362:bool)  [unwired: 1 in]
          n133 = Or(x=w362, y=w373) -> (x .or. y?=w364:bool)
          n134 = case shown="True" w364 {
            tunnel: w385 -> [w422 w432]
            tunnel: [w422 w425] -> w384
            tunnel: w383 -> [_ w427]
            tunnel: w377 -> [_ w428]
            tunnel: w376 -> [_ w430]
            tunnel: w324 -> [_ w431]
            tunnel: w323 -> [_ w424]
            tunnel: w322 -> [_ w423]
            frame False {
            }
            frame True {
              # "Update at 1 Hz"
              n135 = call "Write Single.vim"("Data Element"=w430, "error in"=w432, "Data DVR"=w431) -> ("dup error out"=w429:errorcluster)  [unwired: 8 in]
              n136 = call "Write Single.vim"("Data Element"=w428, "error in"=w429, "Data DVR"=w424) -> ("dup error out"=w426:errorcluster)  [unwired: 8 in]
              n137 = call "Write Single.vim"("Data Element"=w427, "error in"=w426, "Data DVR"=w423) -> ("dup error out"=w425:errorcluster)  [unwired: 8 in]
            }
          }
          n138 = Or(x=w362, y=w378) -> (x .or. y?=w363:bool)
          n139 = global write "Measurements (Global).vi" "ES_2 V Meas"(w331) -> ()
          n140 = global write "Measurements (Global).vi" "ES_2 I Meas"(w330) -> ()
          n141 = global write "Measurements (Global).vi" "ES_2 P Meas"(w326) -> ()
          n142 = global write "Measurements (Global).vi" "ES_2 Q Meas"(w327) -> ()
          n143 = local read "Is VF Device?"() -> (w367:bool)
          n144 = Bundle(cluster=T23 {"DeviceID"="", "SOC (%)"=0.0} ("ES_Measurement"), "DeviceID"=w351, "SOC (%)"=w349) -> (w350:T23)
          n145 = Not(x=w338) -> (.not. x?=w337:bool)
          n146 = Bundle(cluster=T24 {"DeviceID"="", "VFControl"=FALSE, "PControl"=FALSE, "QControl"=FALSE, "PFControl"=FALSE, "PVControl"=FALSE, "Droop"=FALSE, "Unbalanced"=FALSE, "MicrogridVF"=FALSE, "RealDroop(kW)"={"XMin"=0.0, "XMax"=0.0, "YMin"=0.0, "YMax"=0.0}, "ReactiveDroop(kVar)"={"XMin"=0.0, "XMax"=0.0, "YMin"=0.0, "YMax"=0.0}} ("DER_Status"), "DeviceID"=w351, "VFControl"=w338, "PControl"=w337, "QControl"=w337, "PFControl"=w336, "PVControl"=w336, "Droop"=w336, "Unbalanced"=w336, "MicrogridVF"=w367) -> (w381:T24)  [unwired: 2 in]
          n147 = case shown="True" w363 {
            tunnel: w321 -> [_ w419]
            tunnel: w384 -> [w408 w421]
            tunnel: w383 -> [_ w420]
            tunnel: w382 -> [_ w413]
            tunnel: w381 -> [_ w410]
            tunnel: [w408 w409] -> w380
            tunnel: w350 -> [_ w416]
            tunnel: w320 -> [_ w417]
            tunnel: w319 -> [_ w414]
            tunnel: w318 -> [_ w411]
            frame False {
            }
            frame True {
              # "Update at 10 Hz"
              n148 = call "Write Single.vim"("Data Element"=w420, "error in"=w421, "Data DVR"=w419) -> ("dup error out"=w418:errorcluster)  [unwired: 8 in]
              n149 = call "Write Single.vim"("Data Element"=w416, "error in"=w418, "Data DVR"=w417) -> ("dup error out"=w415:errorcluster)  [unwired: 8 in]
              n150 = call "Write Single.vim"("Data Element"=w413, "error in"=w415, "Data DVR"=w414) -> ("dup error out"=w412:errorcluster)  [unwired: 8 in]
              n151 = call "Write Single.vim"("Data Element"=w410, "error in"=w412, "Data DVR"=w411) -> ("dup error out"=w409:errorcluster)  [unwired: 8 in]
            }
          }
          n152 = call <vilib>:"Clear Errors.vi"("error in (no error)"=w380, "specific error code to clear (0: all)"=5038) -> ("error out"=w366:errorcluster, "specific error cleared?"=w361:bool)  [unwired: 4 in]
          n153 = feedback-in #1(w361) -> ()
          n154 = case shown="True" w361 {
            frame False {
            }
            frame True {
              n155 = feedback #2(u32 0 ("5038 Count")) -> (w388:u32)
              n156 = Increment(x=w388) -> (x+1=w389:u32)
              "5038 Count" <- w389
              n157 = feedback-in #2(w389) -> ()
            }
          }
        }
        frame "CheckClose" {
          # "Check to see if MicrogridID has been reset to 0, releasing the device from Microgrid control"
          n158 = Select(t=DDS_State."Close", s=FALSE, f=DDS_State."ReadDDS") -> (s? t:f=w437:T2)
        }
        frame "Close" {
          # "Set MicrogridID to 0 in order for Generation Mode Loop to function correctly."
          # "Deactivate the device"
          # "Release resources associated with microgrid ID, deactivate device, and return to CheckID state"
          n159 = flat-sequence {
            frame #0 {
              # "disables output"
              n160 = local write "Enable INV A"(FALSE ("PWM Enabled")) -> ()
            }
          }
          n161 = local write "MicrogridID"(u8 0 ("MicrogridID")) -> ()
        }
        frame "Shutdown" {
          # "Set MicrogridID to 0 in order for Generation Mode Loop to function correctly."
          # "Deactivate the device"
          # "Release resources and stop loop"
          n162 = flat-sequence {
            frame #0 {
              # "disables output"
              n163 = local write "Enable INV A"(FALSE ("PWM Enabled")) -> ()
            }
          }
          n164 = local write "MicrogridID"(u8 0 ("MicrogridID")) -> ()
        }
      }
      "DDS Loop error out" <- w157
      n165 = global read "Stop (Global).vi" "stop"() -> (w140:bool)
      n166 = local read "MicrogridID"() -> (w144:u8)
      n167 = local read "Is VF Device?"() -> (w143:bool)
      n168 = Unbundle By Name(w157) -> ("status"=→"Error in DDS Loop":bool)
      n169 = local read "DDS State"() -> (w142:T2)
      n170 = Wait (ms)(milliseconds to wait=u32 0) -> (millisecond timer value=w153:u32)
      n171 = Or(x=w140, y=w157) -> (x .or. y?=w159:bool)
      n172 = feedback #3() -> (w152:u32)  [unwired: 1 in]
      n173 = feedback-in #3(w153) -> ()
      n174 = Select(t=DDS_State."Shutdown", s=w159, f=w161) -> (s? t:f=w162:T2)
      n175 = Subtract(x=w153, y=w152) -> (x-y=→"DDS loop time":u32)
      n176 = Bundle("DDS State"=w142, "Is VF Device?"=w143, "MicrogridID"=w144) -> (→"DDS Indicators":T3)  [unwired: 1 in]
      "DDS State" <- w139
    }
    n177 = while "Generation Mode Loop" {
      shift-right: [w51] -> _
      shift-left: w30 -> [w54]
      shift-right: [w45] -> w29
      shift-left: errorcluster {"status"=FALSE, "code"=0, "source"=""} ("error out") -> [w49]
      tunnel: w31 -> [w47]
      tunnel: w23 -> [w50]
      stop <- w44 stop-if-true
      # "Handles generation mode switching"
      n178 = case shown="\"VF Device\"" w54 {
        tunnel: [w56 Generation_Mode_Loop_Selector."Active" w73 w96 Generation_Mode_Loop_Selector."VF Device" Generation_Mode_Loop_Selector."Commissioning" Generation_Mode_Loop_Selector."Commissioning"] -> w52
        tunnel: [_ _ _ _ _ _ TRUE] -> w44
        tunnel: w50 -> [_ _ w69 w93 _ _ _]
        tunnel: w49 -> [w55 w62 w67 w92 w132 w134 w137]
        tunnel: [w55 w62 w66 w91 w132 w134 w137] -> w45
        tunnel: w47 -> [_ _ w68 w86 _ _ _]
        frame "Commissioning" {
          # "Start up case that allows DDS State Machine to get a Microgrid ID before going into rest of state machine"
          n179 = Wait (ms)(milliseconds to wait=u32 100) -> ()  [unwired: 1 out]
          n180 = local read "MicrogridID"() -> (w60:u8)
          n181 = Equal To 0?(x=w60) -> (x = 0?=w59:bool)
          n182 = Select(t=Generation_Mode_Loop_Selector."Commissioning", s=w59, f=Generation_Mode_Loop_Selector."Start") -> (s? t:f=w56:T5)
        }
        frame "Start" {
          # "Initialize reader looking at Generation Mode"
        }
        frame "Active" {
          # "Able to switch generation modes, but not available for VF."
          n183 = Unbundle By Name(w69) -> ("DER_setGenerationMode"=w71:refnum<data-value>)
          n184 = Wait (ms)(milliseconds to wait=u32 100) -> ()  [unwired: 1 out]
          n185 = call "Read Single.vim"("Data Type"=T12 {"DeviceID"="", "Mode"=enum."Invalid"} ("DER_setGenerationMode"), "DeviceID"=w68, "error in"=w67, "Data DVR"=w71) -> ("dup error out"=w66:errorcluster, "Valid"=w64:bool, "Data Element"=w65:T12)  [unwired: 5 in]
          n186 = case shown="True" w64 {
            tunnel: w65 -> [_ w82]
            frame False {
            }
            frame True {
              # "DeviceID Match"
              n187 = Unbundle By Name(w82) -> ("Mode"=w81:T13)
              n188 = case shown="\"VF\"" w81 {
                frame "Invalid", Default {
                }
                frame "PQ" {
                  # "PQ is a valid mode, make sure all settings are correct"
                  n189 = local write "Vf Control"(FALSE ("Vf Control")) -> ()
                }
                frame "VF" {
                  # "Added this case for situation where we hot swap VF devices while offgrid.  If this device is no longer the VF device, it gets kicked to \"Active\" case and setGenerationMode flag is probably still \"VF\""
                  n190 = local write "Vf Control"(FALSE ("Vf Control")) -> ()
                }
                frame "Droop" {
                  n191 = local write "Vf Control"(FALSE ("Vf Control")) -> ()
                }
              }
            }
          }
          n192 = local read "Is VF Device?"() -> (w75:bool)
          n193 = Select(t=Generation_Mode_Loop_Selector."VF Device", s=w75, f=Generation_Mode_Loop_Selector."Active") -> (s? t:f=w74:T5)
          n194 = local read "MicrogridID"() -> (w80:u8)
          n195 = Equal To 0?(x=w80) -> (x = 0?=w79:bool)
          n196 = Select(t=Generation_Mode_Loop_Selector."Close References", s=w79, f=w74) -> (s? t:f=w73:T5)
        }
        frame "VF Device" {
          # "Active, plus available for VF mode.."
          n197 = Unbundle By Name(w93) -> ("DER_setGenerationMode"=w90:refnum<data-value>)
          n198 = Wait (ms)(milliseconds to wait=u32 1) -> ()  [unwired: 1 out]
          n199 = call "Read Single.vim"("Data Type"=T12 {"DeviceID"="", "Mode"=enum."Invalid"} ("DER_setGenerationMode"), "DeviceID"=w86, "error in"=w92, "Data DVR"=w90) -> ("dup error out"=w91:errorcluster, "Valid"=w88:bool, "Data Element"=w87:T12)  [unwired: 5 in]
          n200 = case shown="False" w88 {
            tunnel: w87 -> [_ w120]
            tunnel: [Generation_Mode_Loop_Selector."VF Device" w106] -> w94
            frame False {
              n201 = global read "Measurements (Global).vi" "PCC Status"() -> (w104:bool)
              n202 = Not(x=w104) -> (.not. x?=w103:bool)
              n203 = local write "Vf Control"(w103) -> ()
            }
            frame True {
              # "DeviceID Match"
              n204 = Unbundle By Name(w120) -> ("Mode"=w119:T13)
              n205 = feedback #4() -> (w113:T13)  [unwired: 1 in]
              n206 = case shown="\"VF\"" w119 {
                tunnel: w119 -> [_ w124 w126 w129]
                tunnel: [w121 w124 w126 w129] -> w118
                tunnel: w113 -> [w121 _ _ _]
                frame "Invalid", Default {
                }
                frame "PQ" {
                  # "PQ is a valid mode, make sure all settings are correct"
                  n207 = global read "Measurements (Global).vi" "PCC Status"() -> (w123:bool)
                  n208 = Not(x=w123) -> (.not. x?=w122:bool)
                  n209 = local write "Vf Control"(w122) -> ()
                }
                frame "Droop" {
                  n210 = local write "Vf Control"(FALSE ("Vf Control")) -> ()
                }
                frame "VF" {
                  # "Switches device to Voltage-Frequency control"
                  n211 = global read "Measurements (Global).vi" "PCC Status"() -> (w128:bool)
                  n212 = Not(x=w128) -> (.not. x?=w127:bool)
                  n213 = local write "Vf Control"(w127) -> ()
                }
              }
              n214 = feedback-in #4(w118) -> ()
              n215 = Equal?(x=GenerationMode."PQ", y=w118) -> (x = y?=w115:bool)
              n216 = Equal?(x=GenerationMode."Droop", y=w118) -> (x = y?=w114:bool)
              n217 = Equal?(x=GenerationMode."VF", y=w113) -> (x = y?=w110:bool)
              n218 = Or(x=w115, y=w114) -> (x .or. y?=w111:bool)
              n219 = And(x=w111, y=w110) -> (x .and. y?=w109:bool)
              n220 = Select(t=Generation_Mode_Loop_Selector."Hold", s=w109, f=Generation_Mode_Loop_Selector."VF Device") -> (s? t:f=w106:T5)
            }
          }
          n221 = local read "Is VF Device?"() -> (w98:bool)
          n222 = Select(t=w94, s=w98, f=Generation_Mode_Loop_Selector."Active") -> (s? t:f=w97:T5)
          n223 = local read "MicrogridID"() -> (w102:u8)
          n224 = Equal To 0?(x=w102) -> (x = 0?=w101:bool)
          n225 = Select(t=Generation_Mode_Loop_Selector."Close References", s=w101, f=w97) -> (s? t:f=w96:T5)
        }
        frame "Hold" {
          # "Set P and Q setpoints to current values when transitioning from VF to PQ"
          n226 = local read "Q_meas"() -> (w130:sgl)
          n227 = local read "P_meas"() -> (w131:sgl)
          n228 = local write "P_ref"(w131) -> ()
          n229 = local write "Q_ref"(w130) -> ()
        }
        frame "Close References" {
          # "close connection/reference to DDS Reader for DER_setGenerationMode"
        }
        frame "Shutdown" {
          # "Release resources and close loop"
        }
      }
      "error out GenMode Loop" <- w45
      n230 = Unbundle By Name(w45) -> ("status"=→"Error in Generation Mode Loop":bool)
      n231 = Wait (ms)(milliseconds to wait=u32 0) -> (millisecond timer value=w42:u32)
      n232 = global read "Stop (Global).vi" "stop"() -> (w39:bool)
      n233 = feedback #5() -> (w41:u32)  [unwired: 1 in]
      n234 = feedback-in #5(w42) -> ()
      n235 = Or(x=w45, y=w39) -> (x .or. y?=w48:bool)
      n236 = Subtract(x=w42, y=w41) -> (x-y=→"DDS state m/c loop time":u32)
      n237 = Select(t=Generation_Mode_Loop_Selector."Shutdown", s=w48, f=w52) -> (s? t:f=w51:T5)
    }
    "DeviceID" <- w34
  }
  "Q_ref" <- w6
  "P_ref" <- w7
